vi "Tosca-Wait For Filename.vi"(0 "IPC":T1, 7 "Times out?":bool=TRUE) -> (4 "Filestem":string, 8 "Received":bool, 15 "error out":errorcluster)   [LabVIEW 2020]
uses:
  Tosca-IPC.ctl
  Classes/Parameters/Parameters.lvclass
  Digital Input VIs/Tosca-DI Queue Data.ctl
  Digital Input VIs/Tosca-Input Event.ctl
  Digital Input VIs/Tosca-Input Criterion.ctl
  epl-vi-lib/Utility VIs/Type Defs/Logic State.ctl
  Typedefs/Tosca-Accumulator.ctl
  Typedefs/Tosca-State AODO.ctl
  Typedefs/Tosca-AO Runtime.ctl
  Typedefs/Tosca-DO Runtime.ctl
  epl-vi-lib/Signal Synthesis VIs/4th Generation/Classes/SignalManager/SignalManager.lvclass
  Typedefs/Tosca-Synapse Start Data.ctl
  Tosca-Message.ctl
  Tosca-Message Action.ctl
  Typedefs/Tosca-Thread Type.ctl
  Imaging VIs/Tosca-2P-Notifier Data.ctl
  Typedefs/Tosca-MATLAB Queue Data.ctl
  Visual Stim VIs/Tosca-Grating.ctl
  Visual Stim VIs/Tosca-Grating Type.ctl
  Typedefs/Tosca-File IO Notification.ctl
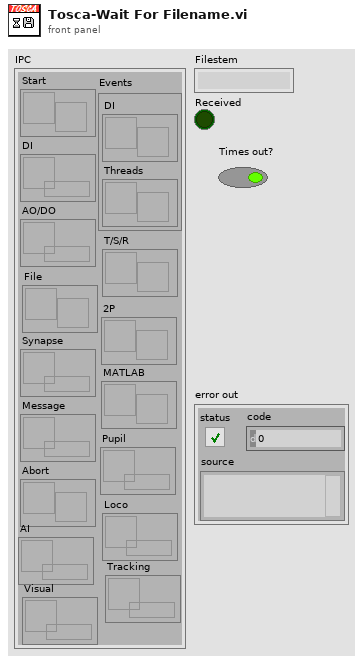
[diagram p1: front panel]
types:
  T1 = typedef "Tosca-IPC.ctl" = cluster{"Start":refnum<notifier>, "DI":refnum<queue>, "AO/DO":refnum<queue>, "Synapse":refnum<queue>, "Message":refnum<queue>, "Abort":refnum<notifier>, "Events":cluster{"DI":refnum<user-event>, "Threads ":refnum<user-event>}, "T/S/R":refnum<notifier>, "2P":refnum<notifier>, "MATLAB":refnum<notifier>, "Pupil":refnum<queue>, "Loco":refnum<queue>, "AI":refnum<queue>, "Tracking":refnum<queue>, "Visual":refnum<queue>, "File":refnum<notifier>}
  T2 = typedef "Tosca-File IO Notification.ctl" = cluster{"Operation":enum16{"Start", "Update", "Finish"}, "Filestem":string}
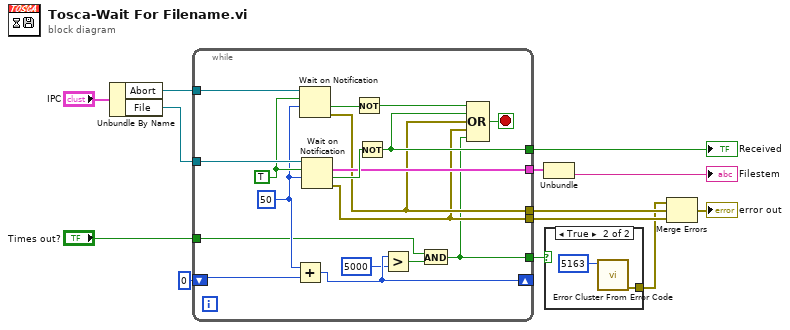
[diagram p0: block diagram]
diagram:
  n1 = Unbundle By Name("IPC") -> ("Abort"=w13:refnum<notifier>, "File"=w12:refnum<notifier>)
  n2 = while {
    tunnel: w13 -> [w30]
    tunnel: w12 -> [w28]
    tunnel: [w25] -> w8
    tunnel: [w24] -> w10
    tunnel: [w23] -> w7
    tunnel: [w22] -> w6
    shift-right: [w18] -> _
    shift-left: 0 -> [w20]
    tunnel: [w15] -> w3
    tunnel: "Times out?" -> [w14]
    stop <- w26 stop-if-true
    w21 = TRUE ("ignore previous (F)")
    w19 = 50 ("timeout in ms (-1)")
    n3 = Add(x=w19, y=w20) -> (x+y=w18:i32)
    n4 = Wait on Notification(notifier=w30, ignore previous (F)=w21, timeout in ms (-1)=w19) -> (timed out?=w31:bool, error out=w23:errorcluster)  [unwired: 1 in, 2 out]
    n5 = Wait on Notification(notifier=w28, ignore previous (F)=w21, timeout in ms (-1)=w19) -> (notification=w24:T2, timed out?=w27:bool, error out=w22:errorcluster)  [unwired: 1 in, 1 out]
    n6 = Not(x=w31) -> (.not. x?=w29:bool)
    n7 = Not(x=w27) -> (.not. x?=w25:bool)
    n8 = Greater?(x=w18, y=5000) -> (0:w16:bool)
    n9 = And(x=w14, y=w16) -> (x .and. y?=w15:bool)
    n10 = Compound Arithmetic op=OR(w29, w25, w23, w22, w15) -> (w26:bool)
  }
  "Received" <- w8
  n11 = Unbundle(w10) -> ("Filestem"=→"Filestem":string)  [unwired: 1 out]
  n12 = case shown="True" w3 {
    tunnel: [_ w33] -> w2
    frame False {
    }
    frame True {
      n13 = call <vilib>:"Error Cluster From Error Code.vi"("error code (0)"=5163) -> ("error out"=w33:errorcluster)  [unwired: 8 in]
    }
  }
  n14 = Merge Errors(w2, w7, w6) -> (→"error out":errorcluster)
